vi "TestPiezo.vi"() -> ()   [LabVIEW 2009]
uses:
  Controls/PIEZO.WAVE.ctl
panel:
  in  "WAVE":T1={"Speed"=0.00017999999999999998, "Stiffness (0.95)"=0.95, "Linear Stroke"=9.999999999999999e-05, "Delay"=0.2} {"Delay" format="%.2f"; "Linear Stroke" format="%.2f"; "Stiffness (0.95)" format="%.2f"; "Speed" format="%.2f"}
  in  "stop":bool
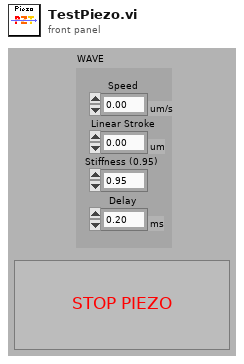
[diagram p1: front panel]
types:
  T1 = typedef "PIEZO.WAVE.ctl" = cluster{"Speed":dbl[unit], "Stiffness (0.95)":dbl, "Linear Stroke":dbl[unit], "Delay":dbl[unit]}
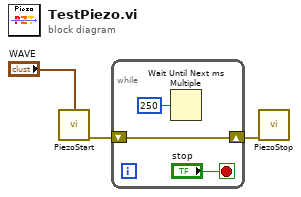
[diagram p0: block diagram]
diagram:
  n1 = call "PiezoStart.vi"("WAVE"="WAVE") -> ("error out"=w3:errorcluster)  [unwired: 8 in]
  n2 = while {
    shift-right: [w5] -> w2
    shift-left: w3 -> [w5]
    stop <- "stop" stop-if-true
    n3 = Wait Until Next ms Multiple(millisecond multiple=u32 250 ("n millisecondes")) -> ()  [unwired: 1 out]
  }
  n4 = call "PiezoStop.vi"("error in (no error)"=w2) -> ()  [unwired: 10 in, 1 out]
